vi "Control Pivot Right.vi"   [LabVIEW 2020]
uses:
  Framework/Robot Global Data.vi
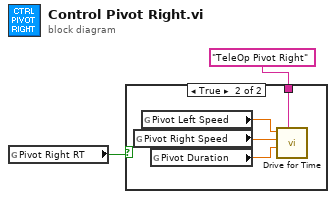
[diagram p0: block diagram]
diagram:
  n1 = global read "Robot Global Data.vi" "Pivot Right RT"() -> (w1:bool)
  n2 = case shown="True" w1 {
    tunnel: "TeleOp Pivot Right" ("Description") -> [_ w6]
    frame False {
    }
    frame True {
      n3 = global read "Robot Global Data.vi" "Pivot Right Speed"() -> (w4:dbl)
      n4 = global read "Robot Global Data.vi" "Pivot Left Speed"() -> (w5:dbl)
      n5 = global read "Robot Global Data.vi" "Pivot Duration"() -> (w3:dbl)
      n6 = call "Drive for Time.vi"("Description"=w6, "Seconds"=w3, "Right Speed"=w4, "Left Speed"=w5) -> ()  [unwired: 7 in, 1 out]
    }
  }
